vi "Is Class Instance.vi"(8 "error in (no error)":errorcluster, 10 "Class Type":enum16{"Project", "Execution", "Step"}(ring), 11 "Control Value":variant) -> (0 "error out":errorcluster, 1 "Class Instance":refnum<class>, 2 "Is Default Value":bool, 3 "Is Class Instance":bool)   [LabVIEW 2015, in "CallVIStep.lvclass"]
uses:
  CallVIStep.lvclass
  Project.lvclass
  Execution.lvclass
  Step.lvclass
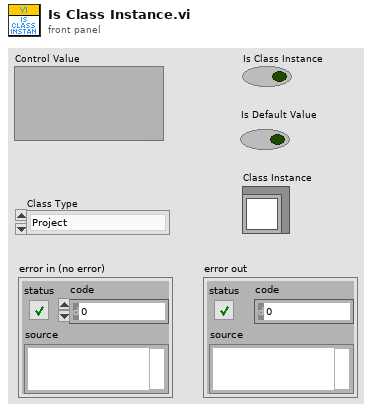
[diagram p1: front panel]
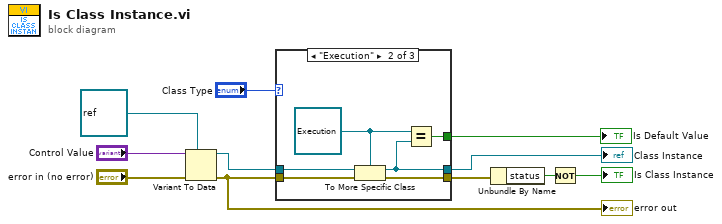
[diagram p0: block diagram]
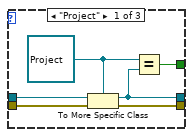
[diagram p2: hidden frame]
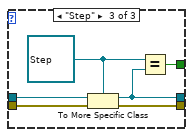
[diagram p3: hidden frame]
diagram:
  n1 = Variant To Data(error in="error in (no error)", type=refnum<class> refnum ("LabVIEW Object"), Variant="Control Value") -> (data=w8:refnum<class>, error out=w7:errorcluster)
  "error out" <- w7
  n2 = case shown="\"Execution\"" "Class Type" {
    tunnel: w8 -> [w17 w23 w29]
    tunnel: w7 -> [w16 w22 w28]
    tunnel: [w15 w21 w27] -> w6
    tunnel: [w14 w18 w25] -> w2
    tunnel: [w12 w20 w26] -> w1
    frame "Project" {
      w13 = refnum<class "Project.lvclass"> refnum ("Project.lvclass")
      n3 = To More Specific Class(target class=w13, reference=w17, error in=w16) -> (specific class reference=w14:refnum<class "Project.lvclass">, error out=w15:errorcluster)
      n4 = Equal?(x=w13, y=w14) -> (x = y?=w12:bool)
    }
    frame "Execution" {
      w19 = refnum<class "Execution.lvclass"> refnum ("Execution.lvclass")
      n5 = To More Specific Class(target class=w19, reference=w23, error in=w22) -> (specific class reference=w18:refnum<class "Execution.lvclass">, error out=w21:errorcluster)
      n6 = Equal?(x=w19, y=w18) -> (x = y?=w20:bool)
    }
    frame "Step" {
      w24 = refnum<class "Step.lvclass"> refnum ("Step.lvclass")
      n7 = To More Specific Class(target class=w24, reference=w29, error in=w28) -> (specific class reference=w25:refnum<class "Step.lvclass">, error out=w27:errorcluster)
      n8 = Equal?(x=w24, y=w25) -> (x = y?=w26:bool)
    }
  }
  "Class Instance" <- w2
  "Is Default Value" <- w1
  n9 = Unbundle By Name(w6) -> ("status"=w5:bool)
  n10 = Not(x=w5) -> (.not. x?=→"Is Class Instance":bool)
